vi "Write TDMS Simple (SubVI).vi"(9 "string":string, 11 "element":waveform(dbl)) -> (0 "error out":errorcluster, 3 "file path out":path)   [LabVIEW 2017]
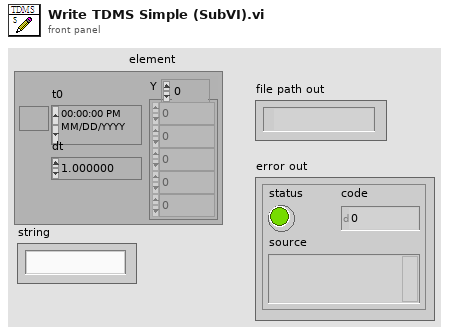
[diagram p1: front panel]
types:
  T1 = enum16{"open", "open or create", "create or replace", "create", "open (read-only)"}
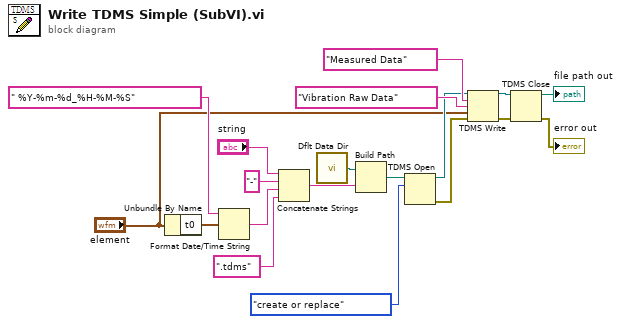
[diagram p0: block diagram]
diagram:
  n1 = Unbundle By Name("element") -> ("t0"=w12:timestamp)
  n2 = Format Date/Time String(time format string (%c)=" %Y-%m-%d_%H-%M-%S", seconds (now)=w12) -> (date/time string=w14:string)  [unwired: 1 in]
  n3 = Concatenate Strings("string", "-" ("string"), w14, ".tdms" ("string")) -> (w19:string)
  n4 = call <vilib>:"Dflt Data Dir.vi"() -> ("App:Default Data Directory"=w5:path)
  n5 = Build Path(base path=w5, name or relative path=w19) -> (appended path=w6:path)
  n6 = TDMS Open(10:T1."create or replace" ("operation (0:open)"), 11:w6) -> (0:w9:errorcluster, 3:w8:refnum<k34>)  [unwired: 5 in]
  n7 = TDMS Write(0:w8, 5:"Measured Data" ("group name in (Untitled)"), 7:"Vibration Raw Data", 9:"element", 11:w9) -> (4:w4:refnum<k34>, 15:w3:errorcluster)  [unwired: 1 in, 2 out]
  n8 = TDMS Close(8:w3, 11:w4) -> (0:→"error out":errorcluster, 3:→"file path out":path)
